vi "ALR init.vi"(8 "error in (no error)":errorcluster, 10 "N_param":i32, 11 "Alarms in":T1) -> (0 "error out":errorcluster, 3 "Alarms out":T1)   [LabVIEW 2019, in "Alarms.lvlib"]
uses:
  Alarms.lvlib
  Ctl/Alarms.ctl
  Ctl/ALR_defs.ctl
  Ctl/ALRs_State.ctl
  Ctl/ALR_ON_OFF.ctl
  Ctl/ALR_Parameters.ctl
  Ctl/ALR code.ctl
  Ctl/ALR type.ctl
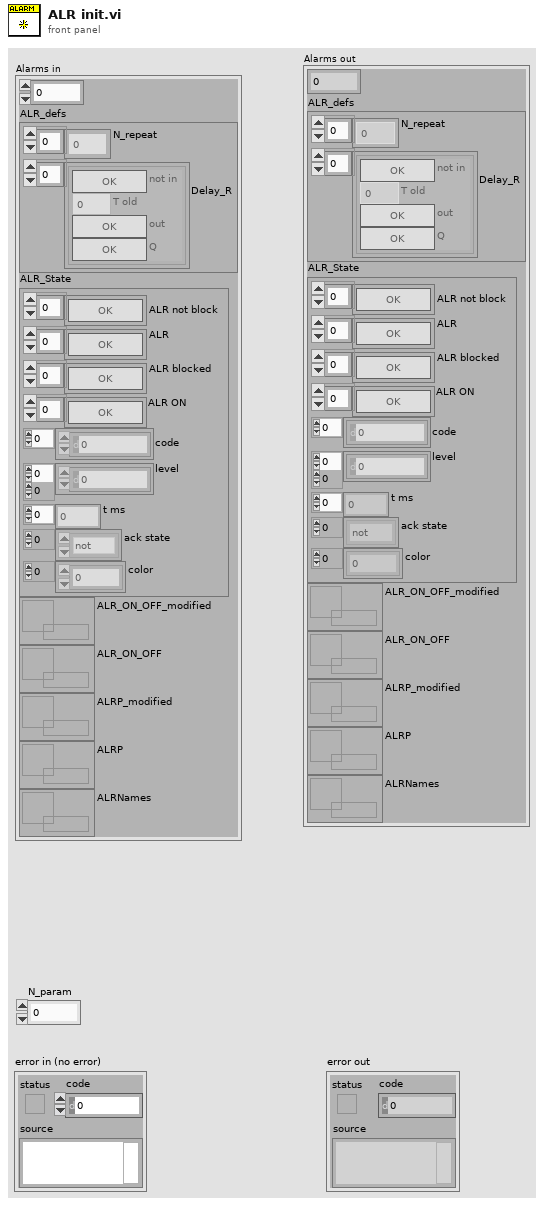
[diagram p1: front panel]
types:
  T1 = typedef "Alarms.lvlib/Alarms.ctl" = cluster{"N_param":i32, "ALR_defs":T2, "ALR_State":T3, "ALR_ON_OFF_modified":refnum<data-value>, "ALR_ON_OFF":refnum<data-value>, "ALRP_modified":refnum<data-value>, "ALRP":refnum<data-value>, "ALRNames":refnum<data-value>}
  T2 = typedef "Alarms.lvlib/ALR_defs.ctl" = cluster{"N_repeat":u32[], "Delay_R":cluster{"not in":bool, "T old":u32, "out":bool, "Q":bool}[]}
  T3 = typedef "Alarms.lvlib/ALRs_State.ctl" = cluster{"ALR not block":bool[], "ALR":bool[], "ALR blocked":bool[], "ALR ON":bool[], "code":i32[], "level":i32[][], "t ms":u32[], "ack state":enum32{"not", "tripped", "reset", "ack"}[], "color":u32[]}
  T4 = typedef "Alarms.lvlib/ALR_ON_OFF.ctl" = cluster{"ALR_ON":bool[], "ALR_OFF":bool[], "ALR_reset":bool[], "ALR_check":bool[], "ALR_block":bool[], "ALR_Ack":bool[]}
  T5 = typedef "Alarms.lvlib/ALR_Parameters.ctl" = cluster{"ALR code":T6[], "ALR type":T7[], "ALRParam":u32[][]}
  T6 = typedef "Alarms.lvlib/ALR code.ctl" = enum16{"CONN", "H", "HH", "L", "LL", "SERR", "ON", "OFF", "XM19", "XM24", "XM47", "XM51", "XM52", "XM53", "XM54", "XM55", "XM56", "XM61", "XM62", "XM63", "XM64", "XM65", "XM66"}
  T7 = typedef "Alarms.lvlib/ALR type.ctl" = enum16{"ACD", "ACDR", "ALRN", "ALR"}
  T8 = cluster{"not in":bool, "T old":u32, "out":bool, "Q":bool}
  T9 = cluster{"not in":bool, "T old":u32, "out":bool, "Q":bool}[]
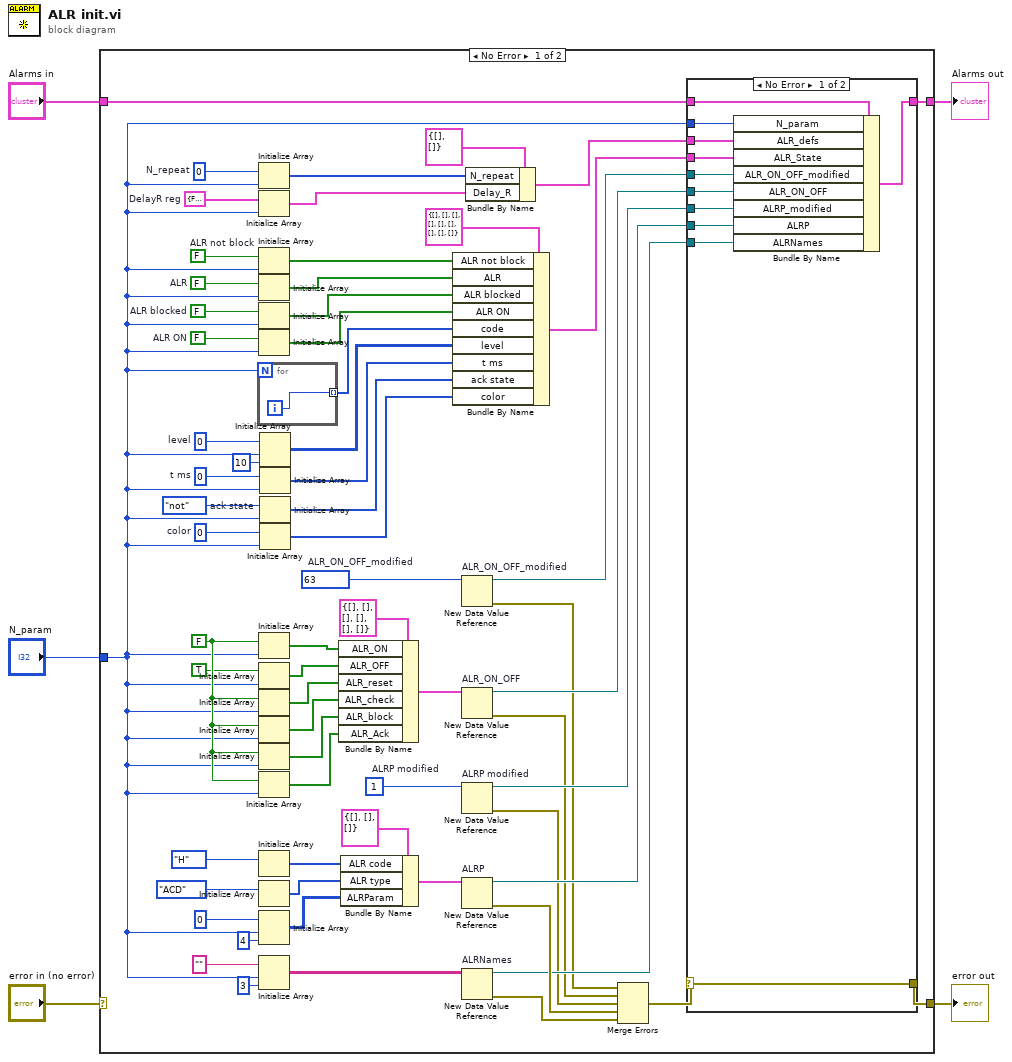
[diagram p0: block diagram]
diagram:
  n1 = case shown="No Error" "error in (no error)" {
    selector: "error in (no error)" -> [_ w85]
    tunnel: [w50 w86] -> w3
    tunnel: "Alarms in" -> [w51 w86]
    tunnel: "N_param" -> [w6 _]
    tunnel: [w48 w85] -> w1
    frame No Error {
      w8 = FALSE  # ALR not block
      w12 = T8 {"not in"=FALSE, "T old"=0, "out"=FALSE, "Q"=FALSE}  # DelayR reg
      w13 = u32 0  # N_repeat
      w20 = u8 1  # ALRP modified
      w25 = u16 63  # ALR_ON_OFF_modified
      w41 = u32 0  # color
      w40 = enum32{"not", "tripped", "reset", "ack"}."not"  # ack state
      w39 = u32 0  # t ms
      w38 = 0  # level
      w44 = FALSE  # ALR ON
      w43 = FALSE  # ALR blocked
      w42 = FALSE  # ALR
      w61 = FALSE ("RS1 Q")
      n2 = for {
        N: w6 -> [_]
        tunnel: [w84] -> w32 mode=indexing
        i -> [w84]
      }
      n3 = Initialize Array(w13, w6) -> (w11:u32[])
      n4 = Initialize Array(w12, w6) -> (w10:T9)
      n5 = Initialize Array(w8, w6) -> (w7:bool[])
      n6 = Initialize Array(w42, w6) -> (w35:bool[])
      n7 = Initialize Array(w43, w6) -> (w34:bool[])
      n8 = Initialize Array(w44, w6) -> (w33:bool[])
      n9 = Initialize Array(w61, w6) -> (w62:bool[])
      n10 = Initialize Array(TRUE ("RS1 Q"), w6) -> (w63:bool[])
      n11 = Initialize Array(w61, w6) -> (w64:bool[])
      n12 = Initialize Array(w61, w6) -> (w65:bool[])
      n13 = Initialize Array(w61, w6) -> (w66:bool[])
      n14 = Initialize Array(w61, w6) -> (w70:bool[])
      n15 = Initialize Array(ALR_code."H" ("ALR code")) -> (w67:T6[])  [unwired: 1 in]
      n16 = Initialize Array(ALR_type."ACD" ("ALR type")) -> (w68:T7[])  [unwired: 1 in]
      n17 = Initialize Array(u32 0 ("ALRParam"), w6, 4 ("dimension size")) -> (w69:u32[][])
      n18 = Initialize Array("" ("ALRNames"), w6, 3 ("dimension size")) -> (w46:string[][])
      n19 = Initialize Array(w38, w6, 10 ("dimension size")) -> (w31:i32[][])
      n20 = Initialize Array(w39, w6) -> (w30:u32[])
      n21 = Initialize Array(w40, w6) -> (w28:enum32{"not", "tripped", "reset", "ack"}[])
      n22 = Initialize Array(w41, w6) -> (w29:u32[])
      n23 = Bundle By Name(cluster=T4 {"ALR_ON"=[], "ALR_OFF"=[], "ALR_reset"=[], "ALR_check"=[], "ALR_block"=[], "ALR_Ack"=[]} ("ALR_ON_OFF"), "ALR_ON"=w62, "ALR_OFF"=w63, "ALR_reset"=w64, "ALR_check"=w65, "ALR_block"=w66, "ALR_Ack"=w70) -> (w49:T4)
      n24 = Bundle By Name(cluster=T5 {"ALR code"=[], "ALR type"=[], "ALRParam"=[]} ("ALRP"), "ALR code"=w67, "ALR type"=w68, "ALRParam"=w69) -> (w47:T5)
      n25 = Bundle By Name(cluster=T3 {"ALR not block"=[], "ALR"=[], "ALR blocked"=[], "ALR ON"=[], "code"=[], "level"=[], "t ms"=[], "ack state"=[], "color"=[]} ("ALR_State"), "ALR not block"=w7, "ALR"=w35, "ALR blocked"=w34, "ALR ON"=w33, "code"=w32, "level"=w31, "t ms"=w30, "ack state"=w28, "color"=w29) -> (w14:T3)
      n26 = New Data Value Reference "ALR_ON_OFF_modified"(data value=w25) -> (data value reference=w21:refnum<data-value>, error out=w18:errorcluster)  [unwired: 1 in]
      n27 = New Data Value Reference "ALR_ON_OFF"(data value=w49) -> (data value reference=w22:refnum<data-value>, error out=w17:errorcluster)  [unwired: 1 in]
      n28 = New Data Value Reference "ALRP modified"(data value=w20) -> (data value reference=w19:refnum<data-value>, error out=w16:errorcluster)  [unwired: 1 in]
      n29 = New Data Value Reference "ALRP"(data value=w47) -> (data value reference=w23:refnum<data-value>, error out=w26:errorcluster)  [unwired: 1 in]
      n30 = New Data Value Reference "ALRNames"(data value=w46) -> (data value reference=w24:refnum<data-value>, error out=w45:errorcluster)  [unwired: 1 in]
      n31 = Bundle By Name(cluster=T2 {"N_repeat"=[], "Delay_R"=[]} ("ALR_defs"), "N_repeat"=w11, "Delay_R"=w10) -> (w9:T2)
      n32 = Merge Errors(w18, w17, w16, w26, w45) -> (w27:errorcluster)
      n33 = case shown="No Error" w27 {
        selector: w27 -> [w77 w82]
        tunnel: w51 -> [w81 w83]
        tunnel: w21 -> [w80 _]
        tunnel: w22 -> [w79 _]
        tunnel: w23 -> [w74 _]
        tunnel: [w78 w83] -> w50
        tunnel: [w77 w82] -> w48
        tunnel: w14 -> [w76 _]
        tunnel: w6 -> [w72 _]
        tunnel: w24 -> [w75 _]
        tunnel: w19 -> [w73 _]
        tunnel: w9 -> [w71 _]
        frame No Error {
          n34 = Bundle By Name(cluster=w81, "N_param"=w72, "ALR_defs"=w71, "ALR_State"=w76, "ALR_ON_OFF_modified"=w80, "ALR_ON_OFF"=w79, "ALRP_modified"=w73, "ALRP"=w74, "ALRNames"=w75) -> (w78:T1)
        }
        frame Error {
        }
      }
    }
    frame Error {
    }
  }
  "error out" <- w1
  "Alarms out" <- w3
